vi "Test U8 Flatten and Unflatten.vi"() -> ()   [LabVIEW 2021]
uses:
  2631624d-cc4e-4626-ba5b-6ee1033d92a5.vi
  8b54960f-aa10-4cd5-858c-4973269b1a77.vi
  d0c9382b-a78e-479c-bfc7-c9ffcc31f28b.vi
  e1924021-44d4-45f9-b731-210da7e63a75.vi
  8a0c8137-5638-4323-b94c-7ef0d8089159.vi
  c1045865-57a9-4a7a-9058-34141a9580d4.vi
  d16bd99d-806c-438b-a2a0-9fff5751a156.vi
  16f3abca-8cc4-4f71-b888-7bdeb5cd89f1.vi
  88f1d4e8-0d26-4b64-adbd-4ba78115a059.vi
  eb70965c-531b-491b-b898-addf9118105b.vi
  3e5bb77c-242d-4622-ad4c-ed122c834b00.vi
  a01e117b-c482-484c-a2ac-20ddba155b86.vi
  a3581276-19ee-4f71-8b5e-94b1362a9c33.vi
  7159e8a4-747c-406e-80f5-7152ae66d07b.vi
  dba2ecab-9623-43f4-b2e0-8813449e1956.vi
  142e2dc9-6fd5-4643-9d5d-299780cc31de.vi
  3ff5cdec-f745-4f13-a5b0-86ed3c89ae69.vi
  2631624d-cc4e-4626-ba5b-6ee1033d92a5.vi/c28b0ead-42ad-4072-80a2-aca7f2bd7ce3.vi
  2631624d-cc4e-4626-ba5b-6ee1033d92a5.vi/48104490-ec73-4168-8754-ff252ec03617.vi
  SubVIs/DataTypes Error.vi
  2631624d-cc4e-4626-ba5b-6ee1033d92a5.vi/543c0f61-77eb-4f29-b175-1688c1700ba4.vi
  8b54960f-aa10-4cd5-858c-4973269b1a77.vi/c28b0ead-42ad-4072-80a2-aca7f2bd7ce3.vi
  8b54960f-aa10-4cd5-858c-4973269b1a77.vi/d83f0d1e-b5f2-409c-a855-55c666a7c55e.vi
  8b54960f-aa10-4cd5-858c-4973269b1a77.vi/c4136907-e772-4046-b7cd-6e4b8d78dccc.vi
  d0c9382b-a78e-479c-bfc7-c9ffcc31f28b.vi/c28b0ead-42ad-4072-80a2-aca7f2bd7ce3.vi
  d0c9382b-a78e-479c-bfc7-c9ffcc31f28b.vi/48104490-ec73-4168-8754-ff252ec03617.vi
  d0c9382b-a78e-479c-bfc7-c9ffcc31f28b.vi/a935433e-9fba-46a4-a99d-56703b8e2dfe.vi
  e1924021-44d4-45f9-b731-210da7e63a75.vi/c28b0ead-42ad-4072-80a2-aca7f2bd7ce3.vi
  e1924021-44d4-45f9-b731-210da7e63a75.vi/d83f0d1e-b5f2-409c-a855-55c666a7c55e.vi
  e1924021-44d4-45f9-b731-210da7e63a75.vi/c4136907-e772-4046-b7cd-6e4b8d78dccc.vi
  8a0c8137-5638-4323-b94c-7ef0d8089159.vi/c28b0ead-42ad-4072-80a2-aca7f2bd7ce3.vi
  8a0c8137-5638-4323-b94c-7ef0d8089159.vi/48104490-ec73-4168-8754-ff252ec03617.vi
  8a0c8137-5638-4323-b94c-7ef0d8089159.vi/a935433e-9fba-46a4-a99d-56703b8e2dfe.vi
  c1045865-57a9-4a7a-9058-34141a9580d4.vi/c28b0ead-42ad-4072-80a2-aca7f2bd7ce3.vi
  c1045865-57a9-4a7a-9058-34141a9580d4.vi/d83f0d1e-b5f2-409c-a855-55c666a7c55e.vi
  c1045865-57a9-4a7a-9058-34141a9580d4.vi/e02991d1-a06a-4e5e-a573-6dce97b92612.vi
  d16bd99d-806c-438b-a2a0-9fff5751a156.vi/c28b0ead-42ad-4072-80a2-aca7f2bd7ce3.vi
  d16bd99d-806c-438b-a2a0-9fff5751a156.vi/48104490-ec73-4168-8754-ff252ec03617.vi
  d16bd99d-806c-438b-a2a0-9fff5751a156.vi/543c0f61-77eb-4f29-b175-1688c1700ba4.vi
  16f3abca-8cc4-4f71-b888-7bdeb5cd89f1.vi/c28b0ead-42ad-4072-80a2-aca7f2bd7ce3.vi
  16f3abca-8cc4-4f71-b888-7bdeb5cd89f1.vi/d83f0d1e-b5f2-409c-a855-55c666a7c55e.vi
  16f3abca-8cc4-4f71-b888-7bdeb5cd89f1.vi/c4136907-e772-4046-b7cd-6e4b8d78dccc.vi
  88f1d4e8-0d26-4b64-adbd-4ba78115a059.vi/c28b0ead-42ad-4072-80a2-aca7f2bd7ce3.vi
  88f1d4e8-0d26-4b64-adbd-4ba78115a059.vi/48104490-ec73-4168-8754-ff252ec03617.vi
  88f1d4e8-0d26-4b64-adbd-4ba78115a059.vi/a935433e-9fba-46a4-a99d-56703b8e2dfe.vi
  eb70965c-531b-491b-b898-addf9118105b.vi/c28b0ead-42ad-4072-80a2-aca7f2bd7ce3.vi
  eb70965c-531b-491b-b898-addf9118105b.vi/d83f0d1e-b5f2-409c-a855-55c666a7c55e.vi
  eb70965c-531b-491b-b898-addf9118105b.vi/e02991d1-a06a-4e5e-a573-6dce97b92612.vi
  3e5bb77c-242d-4622-ad4c-ed122c834b00.vi/c28b0ead-42ad-4072-80a2-aca7f2bd7ce3.vi
  3e5bb77c-242d-4622-ad4c-ed122c834b00.vi/48104490-ec73-4168-8754-ff252ec03617.vi
  3e5bb77c-242d-4622-ad4c-ed122c834b00.vi/543c0f61-77eb-4f29-b175-1688c1700ba4.vi
  a01e117b-c482-484c-a2ac-20ddba155b86.vi/c28b0ead-42ad-4072-80a2-aca7f2bd7ce3.vi
  a01e117b-c482-484c-a2ac-20ddba155b86.vi/d83f0d1e-b5f2-409c-a855-55c666a7c55e.vi
  a01e117b-c482-484c-a2ac-20ddba155b86.vi/e02991d1-a06a-4e5e-a573-6dce97b92612.vi
  a3581276-19ee-4f71-8b5e-94b1362a9c33.vi/c28b0ead-42ad-4072-80a2-aca7f2bd7ce3.vi
  a3581276-19ee-4f71-8b5e-94b1362a9c33.vi/48104490-ec73-4168-8754-ff252ec03617.vi
  a3581276-19ee-4f71-8b5e-94b1362a9c33.vi/543c0f61-77eb-4f29-b175-1688c1700ba4.vi
  7159e8a4-747c-406e-80f5-7152ae66d07b.vi/c28b0ead-42ad-4072-80a2-aca7f2bd7ce3.vi
  7159e8a4-747c-406e-80f5-7152ae66d07b.vi/d83f0d1e-b5f2-409c-a855-55c666a7c55e.vi
  7159e8a4-747c-406e-80f5-7152ae66d07b.vi/e02991d1-a06a-4e5e-a573-6dce97b92612.vi
  dba2ecab-9623-43f4-b2e0-8813449e1956.vi/c28b0ead-42ad-4072-80a2-aca7f2bd7ce3.vi
  dba2ecab-9623-43f4-b2e0-8813449e1956.vi/48104490-ec73-4168-8754-ff252ec03617.vi
  dba2ecab-9623-43f4-b2e0-8813449e1956.vi/543c0f61-77eb-4f29-b175-1688c1700ba4.vi
  142e2dc9-6fd5-4643-9d5d-299780cc31de.vi/c28b0ead-42ad-4072-80a2-aca7f2bd7ce3.vi
  142e2dc9-6fd5-4643-9d5d-299780cc31de.vi/d83f0d1e-b5f2-409c-a855-55c666a7c55e.vi
  142e2dc9-6fd5-4643-9d5d-299780cc31de.vi/c4136907-e772-4046-b7cd-6e4b8d78dccc.vi
  3ff5cdec-f745-4f13-a5b0-86ed3c89ae69.vi/c28b0ead-42ad-4072-80a2-aca7f2bd7ce3.vi
  3ff5cdec-f745-4f13-a5b0-86ed3c89ae69.vi/48104490-ec73-4168-8754-ff252ec03617.vi
  3ff5cdec-f745-4f13-a5b0-86ed3c89ae69.vi/a935433e-9fba-46a4-a99d-56703b8e2dfe.vi
  Errors/Append Error Location.vi
  8b54960f-aa10-4cd5-858c-4973269b1a77.vi/c4136907-e772-4046-b7cd-6e4b8d78dccc.vi/30ec2d62-7bd1-453d-9e4a-daae84816fe3.vi
  8b54960f-aa10-4cd5-858c-4973269b1a77.vi/c4136907-e772-4046-b7cd-6e4b8d78dccc.vi/456025bd-ba3e-42d4-9fa9-b401ab9485ce.vi
  d0c9382b-a78e-479c-bfc7-c9ffcc31f28b.vi/a935433e-9fba-46a4-a99d-56703b8e2dfe.vi/30ec2d62-7bd1-453d-9e4a-daae84816fe3.vi
  d0c9382b-a78e-479c-bfc7-c9ffcc31f28b.vi/a935433e-9fba-46a4-a99d-56703b8e2dfe.vi/456025bd-ba3e-42d4-9fa9-b401ab9485ce.vi
  7159e8a4-747c-406e-80f5-7152ae66d07b.vi/e02991d1-a06a-4e5e-a573-6dce97b92612.vi/30ec2d62-7bd1-453d-9e4a-daae84816fe3.vi
  7159e8a4-747c-406e-80f5-7152ae66d07b.vi/e02991d1-a06a-4e5e-a573-6dce97b92612.vi/456025bd-ba3e-42d4-9fa9-b401ab9485ce.vi
  dba2ecab-9623-43f4-b2e0-8813449e1956.vi/543c0f61-77eb-4f29-b175-1688c1700ba4.vi/30ec2d62-7bd1-453d-9e4a-daae84816fe3.vi
  dba2ecab-9623-43f4-b2e0-8813449e1956.vi/543c0f61-77eb-4f29-b175-1688c1700ba4.vi/456025bd-ba3e-42d4-9fa9-b401ab9485ce.vi
panel:
  out "Pass":bool
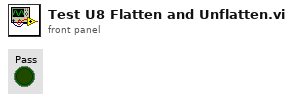
[diagram p1: front panel]
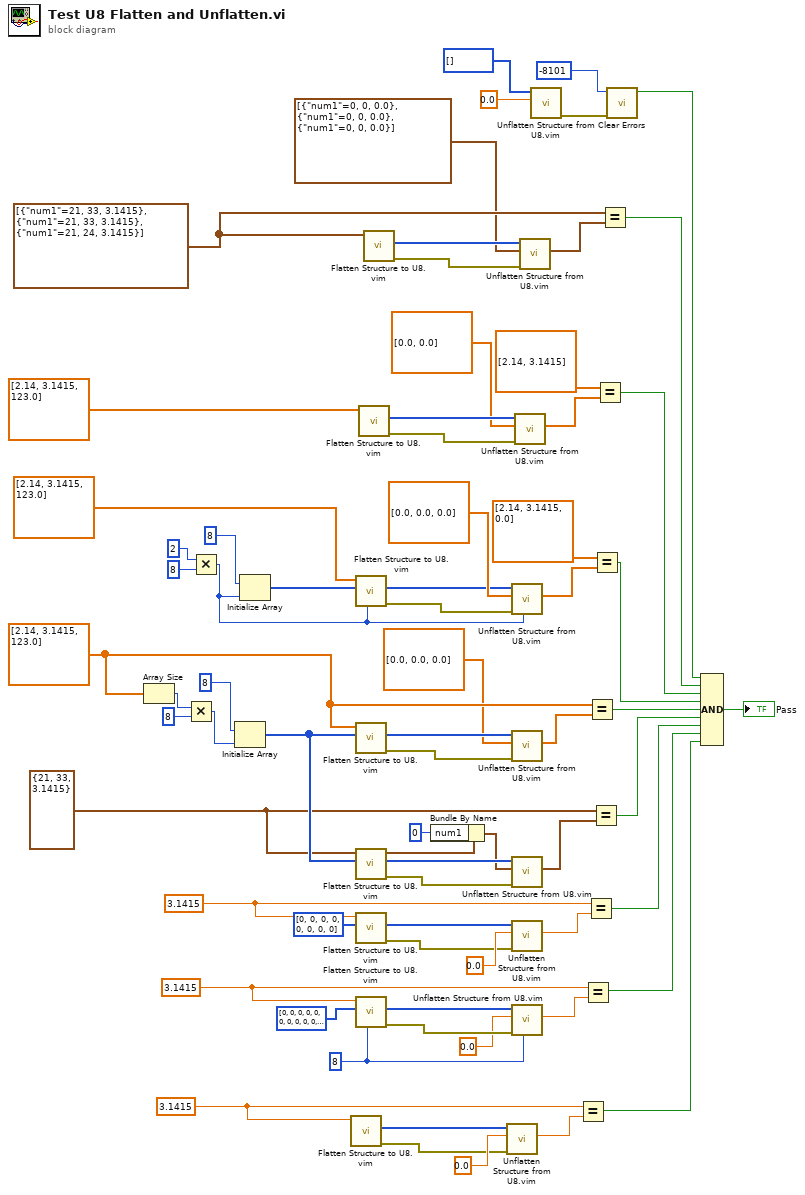
[diagram p0: block diagram]
diagram:
  w8 = cluster{"num1":i64, i64, dbl}[] [{"num1"=21, 33, 3.1415}, {"num1"=21, 33, 3.1415}, {"num1"=21, 24, 3.1415}] ("source")
  w20 = 3.1415
  w38 = u64 8 ("Length override")
  w44 = 3.1415
  w61 = dbl[] [2.14, 3.1415, 123.0] ("source")
  w49 = 3.1415
  w58 = cluster{"num1":i64, i64, dbl} {"num1"=21, 33, 3.1415}
  n1 = Array Size(array=w61) -> (size(s)=w71:i32)
  n2 = Multiply(x=w71, y=8) -> (x*y=w68:i32)
  n3 = Multiply(x=2, y=8) -> (x*y=w27:i32)
  n4 = Initialize Array(u8 8 ("y"), w68) -> (w65:u8[])
  n5 = Initialize Array(u8 8 ("y"), w27) -> (w32:u8[])
  n6 = call "Flatten Structure to U8.vim"("Data to Flatten in"=w20) -> ("error out"=w22:errorcluster, "Flattened Data out"=w24:u8[])  [unwired: 8 in, 1 out]
  n7 = call "Flatten Structure to U8.vim"("Length override"=w27, "Flattened Data in"=w32, "Data to Flatten in"=dbl[] [2.14, 3.1415, 123.0] ("source")) -> ("error out"=w36:errorcluster, "Flattened Data out"=w31:u8[])  [unwired: 6 in, 1 out]
  n8 = call "Flatten Structure to U8.vim"("Flattened Data in"=w65, "Data to Flatten in"=w61) -> ("error out"=w51:errorcluster, "Flattened Data out"=w67:u8[])  [unwired: 7 in, 1 out]
  n9 = call "Flatten Structure to U8.vim"("Flattened Data in"=w65, "Data to Flatten in"=w58) -> ("error out"=w52:errorcluster, "Flattened Data out"=w66:u8[], "Data to Flatten out"=w56:cluster{"num1":i64, i64, dbl})  [unwired: 7 in]
  n10 = call "Flatten Structure to U8.vim"("Flattened Data in"=u8[] [0, 0, 0, 0, 0, 0, 0, 0], "Data to Flatten in"=w49) -> ("error out"=w53:errorcluster, "Flattened Data out"=w64:u8[])  [unwired: 7 in, 1 out]
  n11 = call "Flatten Structure to U8.vim"("Length override"=w38, "Flattened Data in"=u8[] [0, 0, 0, 0, 0, 0, 0, 0, 0, 0, 0, 0, 0, 0, 0, 0], "Data to Flatten in"=w44) -> ("error out"=w42:errorcluster, "Flattened Data out"=w39:u8[])  [unwired: 6 in, 1 out]
  n12 = call "Flatten Structure to U8.vim"("Data to Flatten in"=dbl[] [2.14, 3.1415, 123.0] ("source")) -> ("error out"=w13:errorcluster, "Flattened Data out"=w17:u8[])  [unwired: 8 in, 1 out]
  n13 = call "Flatten Structure to U8.vim"("Data to Flatten in"=w8) -> ("error out"=w11:errorcluster, "Flattened Data out"=w9:u8[])  [unwired: 8 in, 1 out]
  n14 = Bundle By Name(cluster=w56, "num1"=i64 0) -> (w57:cluster{"num1":i64, i64, dbl})
  n15 = call "Unflatten Structure from U8.vim"("error in"=w22, "Type"=0.0, "Flattend Data in"=w24) -> ("Unflattend Data"=w21:dbl)  [unwired: 6 in, 2 out]
  n16 = call "Unflatten Structure from U8.vim"("Length override"=w27, "error in"=w36, "Type"=dbl[] [0.0, 0.0, 0.0] ("source"), "Flattend Data in"=w31) -> ("Unflattend Data"=w33:dbl[])  [unwired: 5 in, 2 out]
  n17 = call "Unflatten Structure from U8.vim"("error in"=w51, "Type"=dbl[] [0.0, 0.0, 0.0] ("source"), "Flattend Data in"=w67) -> ("Unflattend Data"=w62:dbl[])  [unwired: 6 in, 2 out]
  n18 = call "Unflatten Structure from U8.vim"("error in"=w52, "Type"=w57, "Flattend Data in"=w66) -> ("Unflattend Data"=w59:cluster{"num1":i64, i64, dbl})  [unwired: 6 in, 2 out]
  n19 = call "Unflatten Structure from U8.vim"("error in"=w53, "Type"=0.0, "Flattend Data in"=w64) -> ("Unflattend Data"=w50:dbl)  [unwired: 6 in, 2 out]
  n20 = call "Unflatten Structure from U8.vim"("Length override"=w38, "error in"=w42, "Type"=0.0, "Flattend Data in"=w39) -> ("Unflattend Data"=w43:dbl)  [unwired: 5 in, 2 out]
  n21 = call "Unflatten Structure from U8.vim"("error in"=w13, "Type"=dbl[] [0.0, 0.0] ("source"), "Flattend Data in"=w17) -> ("Unflattend Data"=w16:dbl[])  [unwired: 6 in, 2 out]
  n22 = call "Unflatten Structure from U8.vim"("error in"=w11, "Type"=cluster{"num1":i64, i64, dbl}[] [{"num1"=0, 0, 0.0}, {"num1"=0, 0, 0.0}, {"num1"=0, 0, 0.0}] ("source"), "Flattend Data in"=w9) -> ("Unflattend Data"=w10:cluster{"num1":i64, i64, dbl}[])  [unwired: 6 in, 2 out]
  n23 = call "Unflatten Structure from U8.vim"("Type"=0.0, "Flattend Data in"=u8[] []) -> ("error out"=w3:errorcluster)  [unwired: 7 in, 2 out]
  n24 = Equal?(x=w20, y=w21) -> (x = y?=w19:bool)
  n25 = Equal?(x=w44, y=w43) -> (x = y?=w37:bool)
  n26 = Equal?(x=w49, y=w50) -> (x = y?=w46:bool)
  n27 = Equal?(x=w61, y=w62) -> (x = y?=w48:bool)
  n28 = Equal?(x=w58, y=w59) -> (x = y?=w47:bool)
  n29 = Equal?(x=dbl[] [2.14, 3.1415, 0.0] ("source"), y=w33) -> (x = y?=w25:bool)
  n30 = Equal?(x=dbl[] [2.14, 3.1415] ("source"), y=w16) -> (x = y?=w12:bool)
  n31 = Equal?(x=w8, y=w10) -> (x = y?=w7:bool)
  n32 = call <vilib>:"Clear Errors.vi"("error in (no error)"=w3, "specific error code to clear (0: all)"=-8101) -> ("specific error cleared?"=w1:bool)  [unwired: 4 in, 1 out]
  n33 = Compound Arithmetic op=AND(w1, w7, w12, w25, w48, w47, w46, w37, w19) -> (→"Pass":bool)
